vi "FILTER DEAD BAND.vi"(10 "Joystick value in":dbl, 11 "dead band%":dbl=0.1 min=0.04 max=0.75 step=0.01 format="%_3g") -> (3 "Joystick value out":dbl)   [LabVIEW 2020]
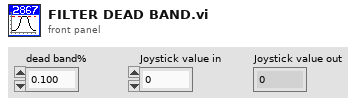
[diagram p1: front panel]
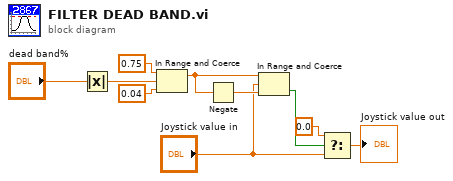
[diagram p0: block diagram]
diagram:
  n1 = Absolute Value(x="dead band%") -> (abs(x)=w4:dbl)
  n2 = In Range and Coerce(upper limit=0.75, x=w4, lower limit=0.04) -> (coerced(x)=w3:dbl)  [unwired: 1 out]
  n3 = Negate(x=w3) -> (-x=w10:dbl)
  n4 = In Range and Coerce(upper limit=w3, x="Joystick value in", lower limit=w10) -> (In Range?=w7:bool)  [unwired: 1 out]
  n5 = Select(t=0.0, s=w7, f="Joystick value in") -> (s? t:f=→"Joystick value out":dbl)
